vi "kalmanGainK.vi"(1 "Pk-1|k-1":T1, 5 "error in (no error)":errorcluster) -> (15 "K gain":T1, 19 "error out":errorcluster)   [LabVIEW 2023, in "Vision.lvclass"]
uses:
  Vision.lvclass
  <vilib>/Analysis/Matrix/Datatypes/RealMatrix.ctl
  <vilib>/Analysis/Matrix/Numeric/Multiply/Multiply - RM,RM.vi
  <vilib>/Analysis/Matrix/Numeric/Add/Add - RM,RM.vi
  <vilib>/Analysis/baseanly.llb/Real Inverse Matrix.vi
  <vilib>/Analysis/Matrix/NI_Matrix.lvlib
  <vilib>/Analysis/NI_AALBase.lvlib
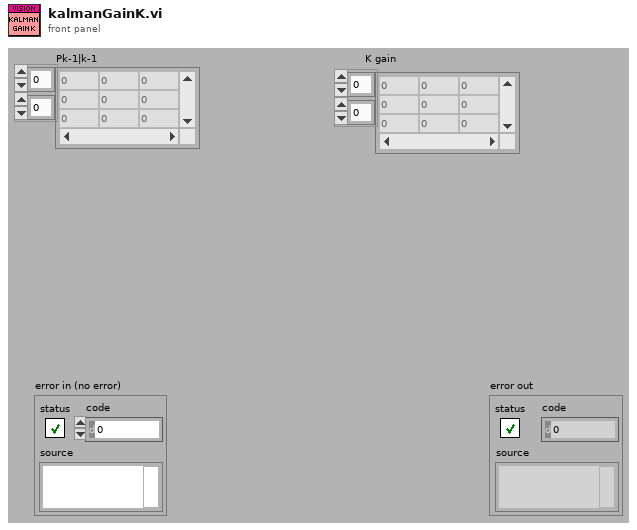
[diagram p1: front panel]
types:
  T1 = typedef "NI_Matrix.lvlib/RealMatrix.ctl" = dbl[][]
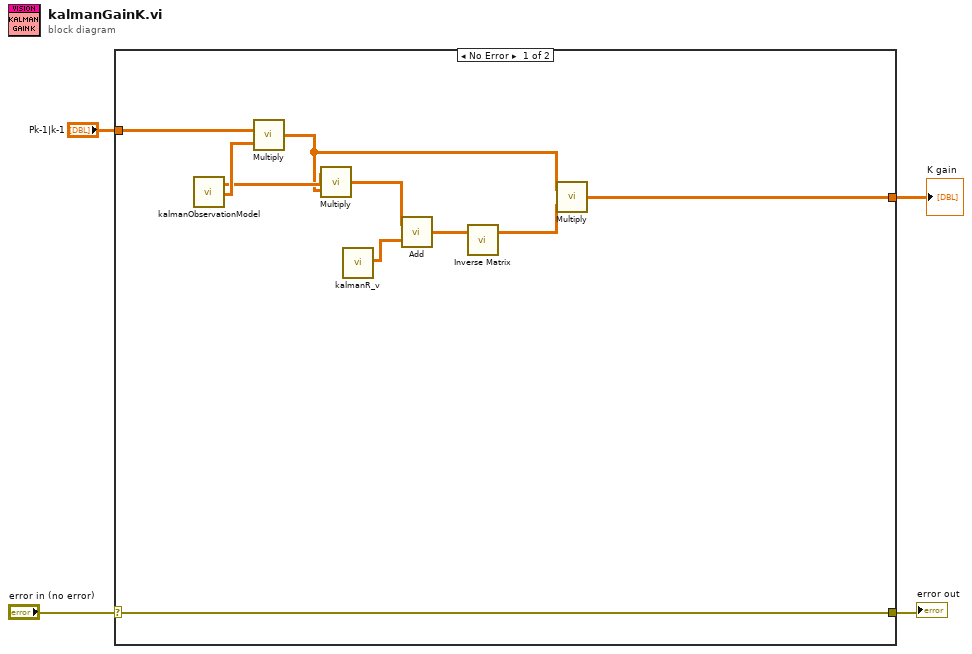
[diagram p0: block diagram]
diagram:
  n1 = case shown="No Error" "error in (no error)" {
    selector: "error in (no error)" -> [w14 w15]
    tunnel: [w14 w15] -> w3
    tunnel: "Pk-1|k-1" -> [w12 _]
    tunnel: [w5 _] -> w1
    frame No Error {
      n2 = call "kalmanObservationModel.vi"() -> ("H"=w11:T1, "H'"=w13:T1)  [unwired: 17 in, 1 out]
      n3 = call-poly <vilib>:"Multiply.vi"("Real Matrix B"=w13, "Real Matrix A"=w12) -> ("A * B"=w7:T1)
      n4 = call-poly <vilib>:"Multiply.vi"("Real Matrix B"=w7, "Real Matrix A"=w11) -> ("A * B"=w10:T1)
      n5 = call "kalmanR_v.vi"() -> ("R_v"=w9:T1)  [unwired: 18 in, 1 out]
      n6 = call-poly <vilib>:"Add.vi"("Real Matrix B"=w9, "Real Matrix A"=w10) -> ("A + B"=w8:T1)
      n7 = call-poly <vilib>:"Inverse Matrix.vi"("Input Matrix"=w8) -> ("Inverse Matrix"=w6:T1)  [unwired: 1 in, 1 out]
      n8 = call-poly <vilib>:"Multiply.vi"("Real Matrix B"=w6, "Real Matrix A"=w7) -> ("A * B"=w5:T1)
    }
    frame Error {
    }
  }
  "error out" <- w3
  "K gain" <- w1
